vi "FreeRTOS.vi"() -> ()   [LabVIEW 2015]
uses:
  <vilib>/Instr/_visa.llb/VISA Configure Serial Port (Instr).vi
panel:
  out "Hight Humidity":bool
  out "Normal Humidity":bool
  out "Lew Humidity":bool
  out "HUMIDITE":dbl(knob) scale=0.0..10.0
  in  "stop":bool
  out "Waveform Chart":dbl(graph)
  out "Humidity Value":string
  in  "VISA resource name":refnum<visa-resource-name>
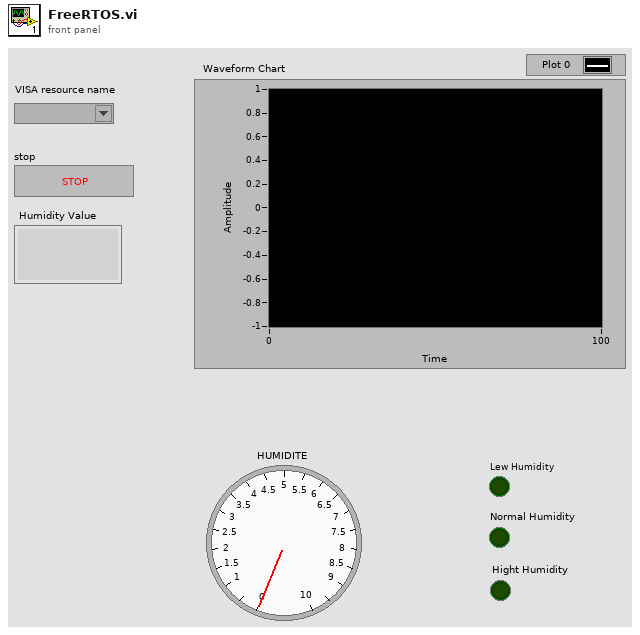
[diagram p1: front panel]
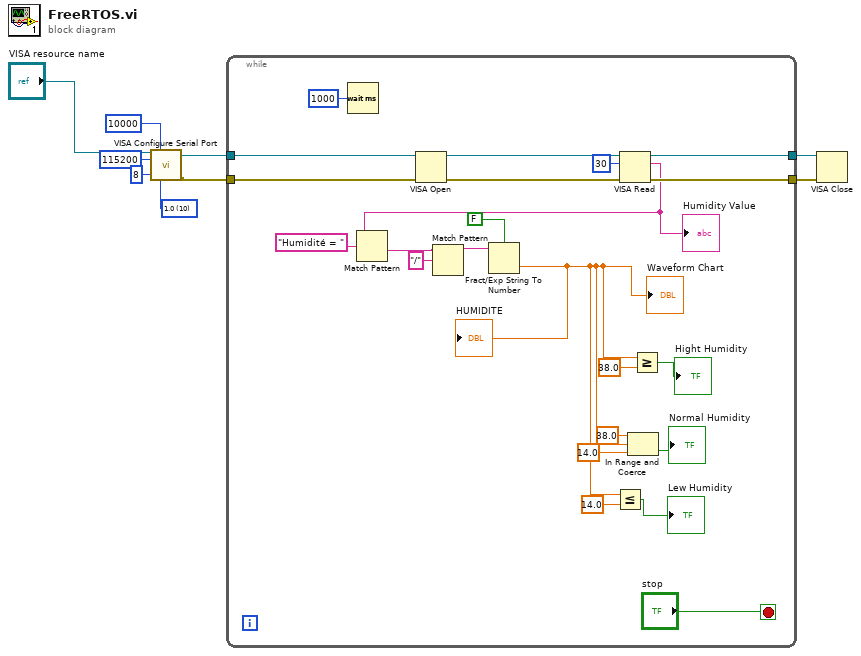
[diagram p0: block diagram]
diagram:
  w3 = u16 10 items=["1.0"=10, "1.5"=15, "2.0"=20] ("stop bits (10: 1 bit)")
  n1 = call-poly "VISA Configure Serial Port"("VISA resource name"="VISA resource name", "timeout (10sec)"=u32 10000, "baud rate (9600)"=u32 115200, "data bits (8)"=u16 8, "stop bits (10: 1 bit)"=w3) -> ("VISA resource name out"=w6:refnum<visa-resource-name>, "error out"=w5:errorcluster)  [unwired: 9 in]
  n2 = while {
    tunnel: [w31] -> w8
    tunnel: [w29] -> w7
    tunnel: w6 -> [w28]
    tunnel: w5 -> [w27]
    stop <- "stop" stop-if-true
    n3 = Wait (ms)(milliseconds to wait=u32 1000) -> ()  [unwired: 1 out]
    n4 = VISA Open(error in (no error)=w27, VISA resource name=w28) -> (VISA resource name=w32:refnum<visa-resource-name>, error out=w30:errorcluster)  [unwired: 3 in]
    n5 = VISA Read(VISA resource name=w32, byte count=u32 30, error in (no error)=w30) -> (VISA resource name out=w31:refnum<visa-resource-name>, read buffer=w24:string, error out=w29:errorcluster)  [unwired: 1 out]
    "Humidity Value" <- w24
    n6 = Match Pattern(string=w24, regular expression="Humidité = " ("text")) -> (after substring=w22:string)  [unwired: 1 in, 3 out]
    n7 = Match Pattern(string=w22, regular expression="/") -> (before substring=w20:string)  [unwired: 1 in, 3 out]
    n8 = Fract/Exp String To Number(use system decimal point (T)=FALSE, string=w20) -> (number=w10:dbl)  [unwired: 2 in, 1 out]
    "Waveform Chart" <- w10
    "HUMIDITE" <- w10
    n9 = Less Or Equal?(x=w10, y=14.0) -> (x <= y?=→"Lew Humidity":bool)
    n10 = In Range and Coerce(upper limit=38.0, x=w10, lower limit=14.0) -> (In Range?=→"Normal Humidity":bool)  [unwired: 1 out]
    n11 = Greater Or Equal?(x=w10, y=38.0) -> (x >= y?=→"Hight Humidity":bool)
  }
  n12 = VISA Close(VISA resource name=w8, error in (no error)=w7) -> ()  [unwired: 1 out]
